vi "DRIVE_STRAIGHT_POWER.vi"(10 "argv":string[](array[string]), 11 "args":u8) -> ()   [LabVIEW 2015]
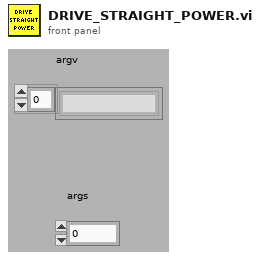
[diagram p1: front panel]
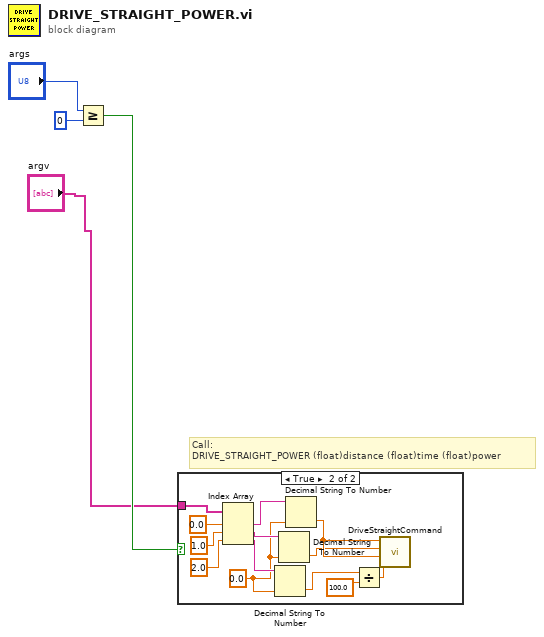
[diagram p0: block diagram]
diagram:
  # "Call:\nDRIVE_STRAIGHT_POWER (float)distance (float)time (float)power"
  n1 = Greater Or Equal?(x="args", y=u8 0) -> (x >= y?=w4:bool)
  n2 = case shown="True" w4 {
    tunnel: "argv" -> [_ w13]
    frame False {
    }
    frame True {
      w8 = 0.0
      n3 = Index Array(array=w13, index #1=0.0 ("default (0 I32)"), index #2=1.0 ("default (0 I32)"), index #3=2.0) -> (element #1=w15:string, element #2=w14:string, element #3=w10:string)
      n4 = Decimal String To Number(string=w10, default (0L)=w8) -> (number=w6:dbl)  [unwired: 1 in, 1 out]
      n5 = Decimal String To Number(string=w14, default (0L)=w8) -> (number=w11:dbl)  [unwired: 1 in, 1 out]
      n6 = Decimal String To Number(string=w15, default (0L)=w8) -> (number=w12:dbl)  [unwired: 1 in, 1 out]
      n7 = Divide(x=w6, y=100.0) -> (x/y=w5:dbl)
      n8 = call "DriveStraightCommand.vi"("speed"=w5, "Fwd Bwd"=w12, "Delay ms"=w11, "distance"=w12) -> ()  [unwired: 8 in]
    }
  }
